vi "Read Channel Specification.vi"(8 "error in (no error)":errorcluster, 11 "FixedChannelTBModuleDecideFeatures in":refnum<class "FixedChannelTBModuleDecideFeatures.lvclass">) -> (0 "error out":errorcluster, 2 "Channel Specification":T1[](array[typedef]), 3 "FixedChannelTBModuleDecideFeatures out":refnum<class "FixedChannelTBModuleDecideFeatures.lvclass">)   [LabVIEW 2013, in "FixedChannelTBModuleDecideFeatures.lvclass"]
uses:
  FixedChannelTBModuleDecideFeatures.lvclass
  channel configuration.ctl
  <vilib>/NI/Tag Bus Module Framework/channel/channel classification.ctl
  <vilib>/NI/Tag Bus/tag/Data Type.ctl
  FixedChannelTBModuleDecideFeatures.lvclass/FixedChannelTBModuleDecideFeatures.ctl
  <vilib>/NI/Tag Bus Module Framework/channel/TBM channel.lvclass
  <vilib>/NI/Tag Bus/tag/tag descriptor.lvclass
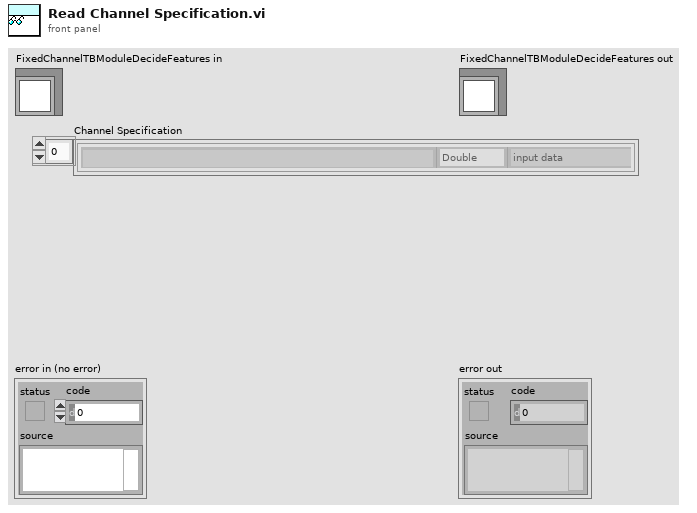
[diagram p1: front panel]
types:
  T1 = typedef "FixedChannelTBModuleDecideFeatures.lvclass/channel configuration.ctl" = cluster{"Name":string, "channel classification":T2, "data type":T3}
  T2 = typedef "TBM channel.lvclass/channel classification.ctl" = enum16{"input data", "output data", "processing parameter", "processing result"}
  T3 = typedef "tag bus.lvlib/tag descriptor.lvclass/Data Type.ctl" = enum16{"Double", "Single", "I64", "I32", "I16", "I8", "U64", "U32", "U16", "U8", "Boolean", "String", "Array of Double", "Array of Single", "Array of I64", "Array of I32", "Array of I16", "Array of I8", "Array of U64", "Array of U32", "Array of U16", "Array of U8", "Array of Boolean", "Array of String"}
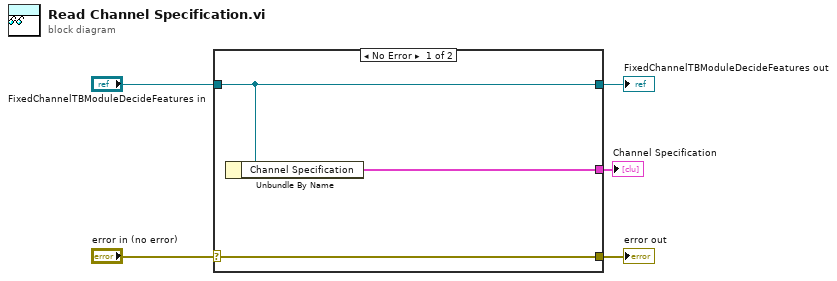
[diagram p0: block diagram]
diagram:
  n1 = case shown="No Error" "error in (no error)" {
    selector: "error in (no error)" -> [w8 w9]
    tunnel: [w8 w9] -> w4
    tunnel: [w7 w10] -> w2
    tunnel: "FixedChannelTBModuleDecideFeatures in" -> [w7 w10]
    tunnel: [w6 _] -> w1
    frame No Error {
      n2 = Unbundle By Name(w7) -> ("Channel Specification"=w6:T1[])
    }
    frame Error {
    }
  }
  "error out" <- w4
  "FixedChannelTBModuleDecideFeatures out" <- w2
  "Channel Specification" <- w1
